vi "SynapseAPI-Set Subject (create).vi"(0 "URL":string="http://localhost:24414", 7 "subject":string, 11 "error in (no error)":errorcluster) -> (15 "error out":errorcluster)   [LabVIEW 2020]
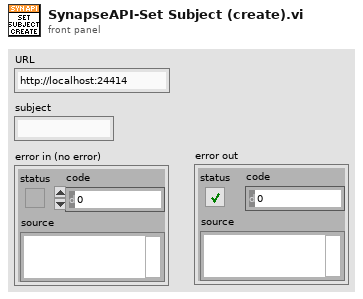
[diagram p1: front panel]
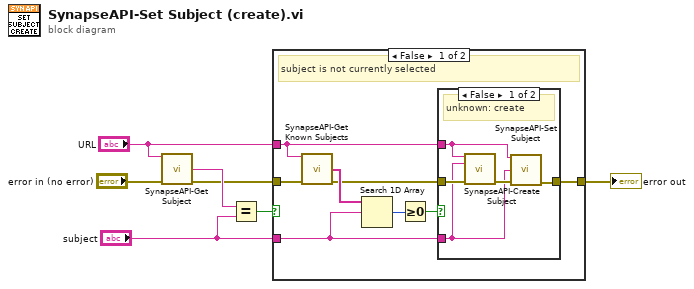
[diagram p0: block diagram]
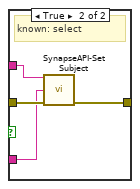
[diagram p2: hidden frame]
diagram:
  n1 = call "SynapseAPI-Get Subject.vi"("URL"="URL", "error in (no error)"="error in (no error)") -> ("subject"=w6:string, "error out"=w4:errorcluster)  [unwired: 12 in]
  n2 = Equal?(x=w6, y="subject") -> (x = y?=w5:bool)
  n3 = case shown="False" w5 {
    tunnel: w4 -> [w15 w25]
    tunnel: "URL" -> [w11 _]
    tunnel: "subject" -> [w8 _]
    tunnel: [w9 w25] -> w1
    frame False {
      # "subject is not currently selected"
      n4 = call "SynapseAPI-Get Known Subjects.vi"("URL"=w11, "error in (no error)"=w15) -> ("subjects"=w14:string[], "error out"=w10:errorcluster)  [unwired: 12 in]
      n5 = Search 1D Array(1D array=w14, element=w8) -> (index of element=w13:i32)  [unwired: 1 in]
      n6 = Greater Or Equal To 0?(x=w13) -> (x >= 0?=w12:bool)
      n7 = case shown="False" w12 {
        tunnel: w11 -> [w18 w23]
        tunnel: w10 -> [w20 w24]
        tunnel: [w17 w22] -> w9
        tunnel: w8 -> [w16 w21]
        frame False {
          # "unknown: create"
          n8 = call "SynapseAPI-Create Subject.vi"("URL"=w18, "subject"=w16, "error in (no error)"=w20) -> ("error out"=w19:errorcluster)  [unwired: 12 in]
          n9 = call "SynapseAPI-Set Subject.vi"("URL"=w18, "subject"=w16, "error in (no error)"=w19) -> ("error out"=w17:errorcluster)  [unwired: 12 in]
        }
        frame True {
          # "known: select"
          n10 = call "SynapseAPI-Set Subject.vi"("URL"=w23, "subject"=w21, "error in (no error)"=w24) -> ("error out"=w22:errorcluster)  [unwired: 12 in]
        }
      }
    }
    frame True {
    }
  }
  "error out" <- w1
